vi "read gain.vi"() -> ()   [LabVIEW 2009]
panel:
  out "Read buffer after RDA removal":string
  out "Read buffer coming directly from VI":string
  out "Gain Read (After formatted to number)":dbl
  out "error out":errorcluster
  out "VISA resource name out":refnum<visa-resource-name>
  in  "error in (no error)":errorcluster
  in  "VISA resource name":refnum<visa-resource-name>="GPIB0::12::INSTR"
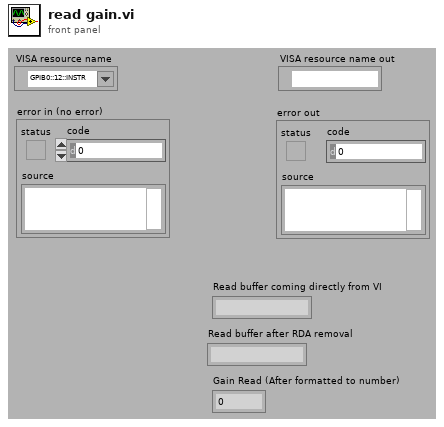
[diagram p1: front panel]
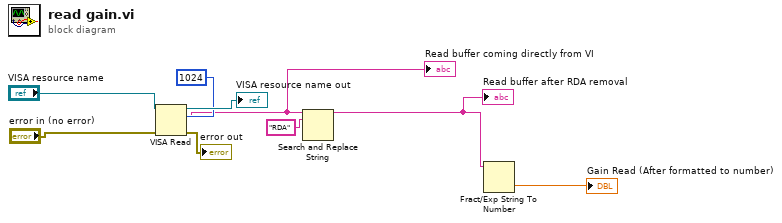
[diagram p0: block diagram]
diagram:
  n1 = VISA Read(VISA resource name="VISA resource name", byte count=u32 1024, error in (no error)="error in (no error)") -> (VISA resource name out=→"VISA resource name out":refnum<visa-resource-name>, read buffer=w2:string, error out=→"error out":errorcluster)  [unwired: 1 out]
  "Read buffer coming directly from VI" <- w2
  n2 = Search and Replace String(input string=w2, search string="RDA") -> (result string=w1:string)  [unwired: 6 in, 3 out]
  "Read buffer after RDA removal" <- w1
  n3 = Fract/Exp String To Number(string=w1) -> (number=→"Gain Read (After formatted to number)":dbl)  [unwired: 3 in, 1 out]
